vi "gantry移動定位_六邊形(內切圓)(旋轉).vi"() -> ()   [LabVIEW 2016]
uses:
  Classes/Controller/Motion/A3200 Folder/A3200.lvclass
panel:
  out "z":dbl
  in  "旋轉角度":dbl
  out "點座標":dbl[][](array[numeric])
  in  "內切圓半徑":dbl=100.0
  in  "中心點座標":dbl[](array[numeric])
  out "Final Position":dbl[](array[numeric])
  out "Initial position":dbl[](array[numeric])
  in  "Speed (mm/s)":dbl=40.0
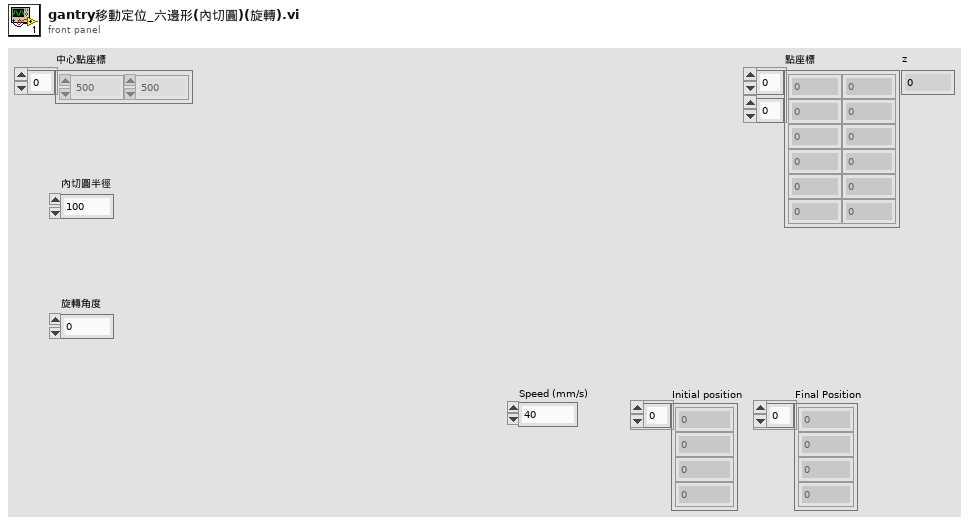
[diagram p1: front panel]
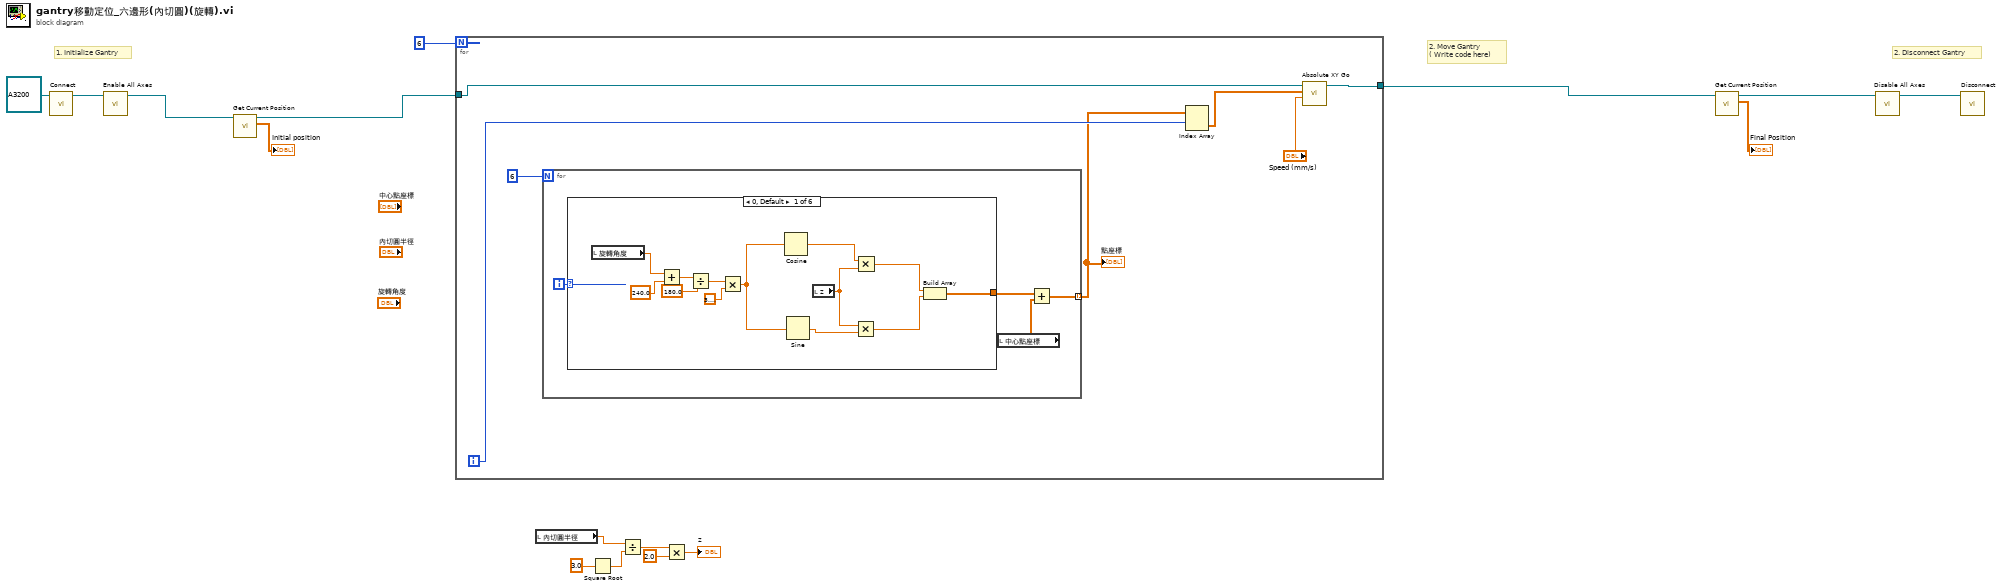
[diagram p0: block diagram]
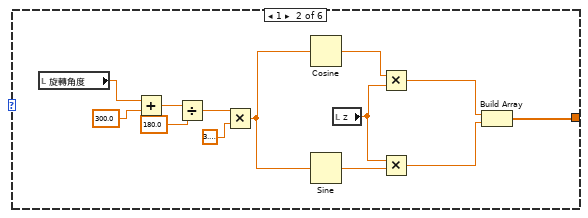
[diagram p2: hidden frame]
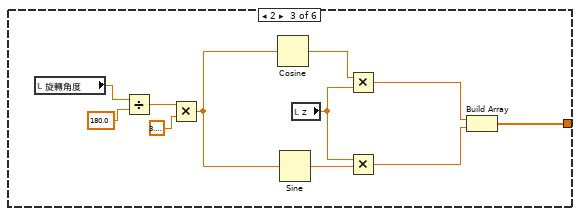
[diagram p3: hidden frame]
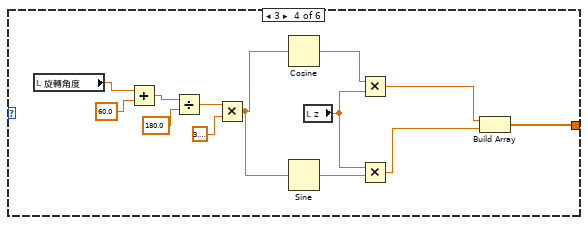
[diagram p4: hidden frame]
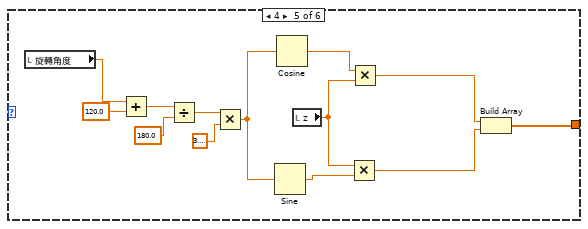
[diagram p5: hidden frame]
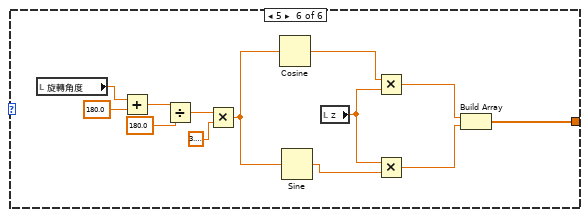
[diagram p6: hidden frame]
diagram:
  # "1. Initialize Gantry"
  # "2. Disconnect Gantry"
  # "2. Move Gantry \n( Write code here)"
  n1 = call-dynamic "Connect.vi"("Gantry in"=refnum<class "A3200.lvclass"> refnum ("A3200.lvclass")) -> ("Gantry out"=w11:refnum<class "A3200.lvclass">)  [unwired: 9 in, 1 out]
  n2 = call-dynamic "Enable All Axes.vi"("A3200 in"=w11) -> ("A3200 out"=w10:refnum<class "A3200.lvclass">)  [unwired: 9 in, 1 out]
  n3 = call-dynamic "Get Current Position.vi"("Gantry in"=w10) -> ("XYZTheta Out"=→"Initial position":dbl[], "Gantry out"=w9:refnum<class "A3200.lvclass">)  [unwired: 8 in, 1 out]
  n4 = for {
    N: 6 -> [_]
    tunnel: w9 -> [w21]
    tunnel: [w20] -> w8
    i -> [w23]
    n5 = for {
      N: 6 -> [_]
      tunnel: [w25] -> w18 mode=indexing
      i -> [w27]
      n6 = case shown="0, Default" w27 {
        tunnel: [w40 w41 w54 w65 w78 w103] -> w24
        frame 0, Default {
          n7 = local read "旋轉角度"() -> (w39:dbl)
          n8 = Add(x=w39, y=240.0) -> (x+y=w37:dbl)
          n9 = Divide(x=w37, y=180.0) -> (x/y=w35:dbl)
          n10 = Multiply(x=w35, y=3.141592653589793) -> (x*y=w31:dbl)
          n11 = Cosine(x=w31) -> (cos(x)=w33:dbl)
          n12 = Sine(x=w31) -> (sin(x)=w30:dbl)
          n13 = local read "z"() -> (w29:dbl)
          n14 = Multiply(x=w29, y=w30) -> (x*y=w28:dbl)
          n15 = Multiply(x=w33, y=w29) -> (x*y=w32:dbl)
          n16 = Build Array(w32, w28) -> (w40:dbl[])
        }
        frame 1 {
          n17 = local read "旋轉角度"() -> (w53:dbl)
          n18 = Add(x=w53, y=300.0) -> (x+y=w51:dbl)
          n19 = Divide(x=w51, y=180.0) -> (x/y=w49:dbl)
          n20 = Multiply(x=w49, y=3.141592653589793) -> (x*y=w45:dbl)
          n21 = Cosine(x=w45) -> (cos(x)=w47:dbl)
          n22 = Sine(x=w45) -> (sin(x)=w44:dbl)
          n23 = local read "z"() -> (w43:dbl)
          n24 = Multiply(x=w47, y=w43) -> (x*y=w46:dbl)
          n25 = Multiply(x=w43, y=w44) -> (x*y=w42:dbl)
          n26 = Build Array(w46, w42) -> (w41:dbl[])
        }
        frame 2 {
          n27 = local read "旋轉角度"() -> (w64:dbl)
          n28 = Divide(x=w64, y=180.0) -> (x/y=w62:dbl)
          n29 = Multiply(x=w62, y=3.141592653589793) -> (x*y=w59:dbl)
          n30 = Cosine(x=w59) -> (cos(x)=w60:dbl)
          n31 = Sine(x=w59) -> (sin(x)=w58:dbl)
          n32 = local read "z"() -> (w57:dbl)
          n33 = Multiply(x=w60, y=w57) -> (x*y=w56:dbl)
          n34 = Multiply(x=w57, y=w58) -> (x*y=w55:dbl)
          n35 = Build Array(w56, w55) -> (w54:dbl[])
        }
        frame 3 {
          n36 = local read "旋轉角度"() -> (w77:dbl)
          n37 = Add(x=w77, y=60.0) -> (x+y=w75:dbl)
          n38 = Divide(x=w75, y=180.0) -> (x/y=w73:dbl)
          n39 = Multiply(x=w73, y=3.141592653589793) -> (x*y=w70:dbl)
          n40 = Cosine(x=w70) -> (cos(x)=w71:dbl)
          n41 = Sine(x=w70) -> (sin(x)=w69:dbl)
          n42 = local read "z"() -> (w68:dbl)
          n43 = Multiply(x=w71, y=w68) -> (x*y=w67:dbl)
          n44 = Multiply(x=w68, y=w69) -> (x*y=w66:dbl)
          n45 = Build Array(w67, w66) -> (w65:dbl[])
        }
        frame 4 {
          n46 = local read "旋轉角度"() -> (w90:dbl)
          n47 = Add(x=w90, y=120.0) -> (x+y=w88:dbl)
          n48 = Divide(x=w88, y=180.0) -> (x/y=w86:dbl)
          n49 = Multiply(x=w86, y=3.141592653589793) -> (x*y=w83:dbl)
          n50 = Sine(x=w83) -> (sin(x)=w82:dbl)
          n51 = Cosine(x=w83) -> (cos(x)=w84:dbl)
          n52 = local read "z"() -> (w81:dbl)
          n53 = Multiply(x=w81, y=w82) -> (x*y=w79:dbl)
          n54 = Multiply(x=w84, y=w81) -> (x*y=w80:dbl)
          n55 = Build Array(w80, w79) -> (w78:dbl[])
        }
        frame 5 {
          n56 = local read "旋轉角度"() -> (w102:dbl)
          n57 = Add(x=w102, y=180.0) -> (x+y=w100:dbl)
          n58 = Divide(x=w100, y=180.0) -> (x/y=w98:dbl)
          n59 = Multiply(x=w98, y=3.141592653589793) -> (x*y=w94:dbl)
          n60 = Cosine(x=w94) -> (cos(x)=w96:dbl)
          n61 = Sine(x=w94) -> (sin(x)=w93:dbl)
          n62 = local read "z"() -> (w92:dbl)
          n63 = Multiply(x=w96, y=w92) -> (x*y=w95:dbl)
          n64 = Multiply(x=w92, y=w93) -> (x*y=w91:dbl)
          n65 = Build Array(w95, w91) -> (w103:dbl[])
        }
      }
      n66 = local read "中心點座標"() -> (w26:dbl[])
      n67 = Add(x=w24, y=w26) -> (x+y=w25:dbl[])
    }
    "點座標" <- w18
    n68 = Index Array(array=w18, index (row)=w23) -> (element=w17:dbl[])  [unwired: 1 in]
    n69 = call-dynamic "Absolute XY Go.vi"("Speed"="Speed (mm/s)", "XY"=w17, "Gantry in"=w21) -> ("Gantry out"=w20:refnum<class "A3200.lvclass">)  [unwired: 7 in, 1 out]
  }
  n70 = local read "內切圓半徑"() -> (w6:dbl)
  n71 = Square Root(x=3.0) -> (sqrt(x)=w4:dbl)
  n72 = Divide(x=w6, y=w4) -> (x/y=w3:dbl)
  n73 = Multiply(x=w3, y=2.0) -> (x*y=→"z":dbl)
  n74 = call-dynamic "Get Current Position.vi"("Gantry in"=w8) -> ("XYZTheta Out"=→"Final Position":dbl[], "Gantry out"=w14:refnum<class "A3200.lvclass">)  [unwired: 8 in, 1 out]
  n75 = call-dynamic "Disable All Axes.vi"("Gantry in"=w14) -> ("Gantry out"=w15:refnum<class "A3200.lvclass">)  [unwired: 9 in, 1 out]
  n76 = call-dynamic "Disconnect.vi"("Gantry in"=w15) -> ()  [unwired: 9 in, 1 out]
